vi "test_CalculateSpecificationBuildOrder.vi"() -> (3 "Pass?":bool)   [LabVIEW 2020, in "Tests.SolutionBuilder.lvlib"]
uses:
  Tests.SolutionBuilder.lvlib
  SolutionBuilder/SolutionBuilder.lvclass
  SolutionBuilder/ProjectItem/ProjectItem.lvclass
panel:
  out "test results":u32 format="%02b"
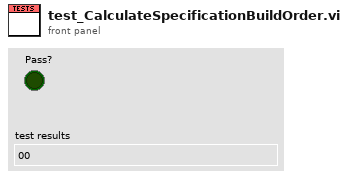
[diagram p1: front panel]
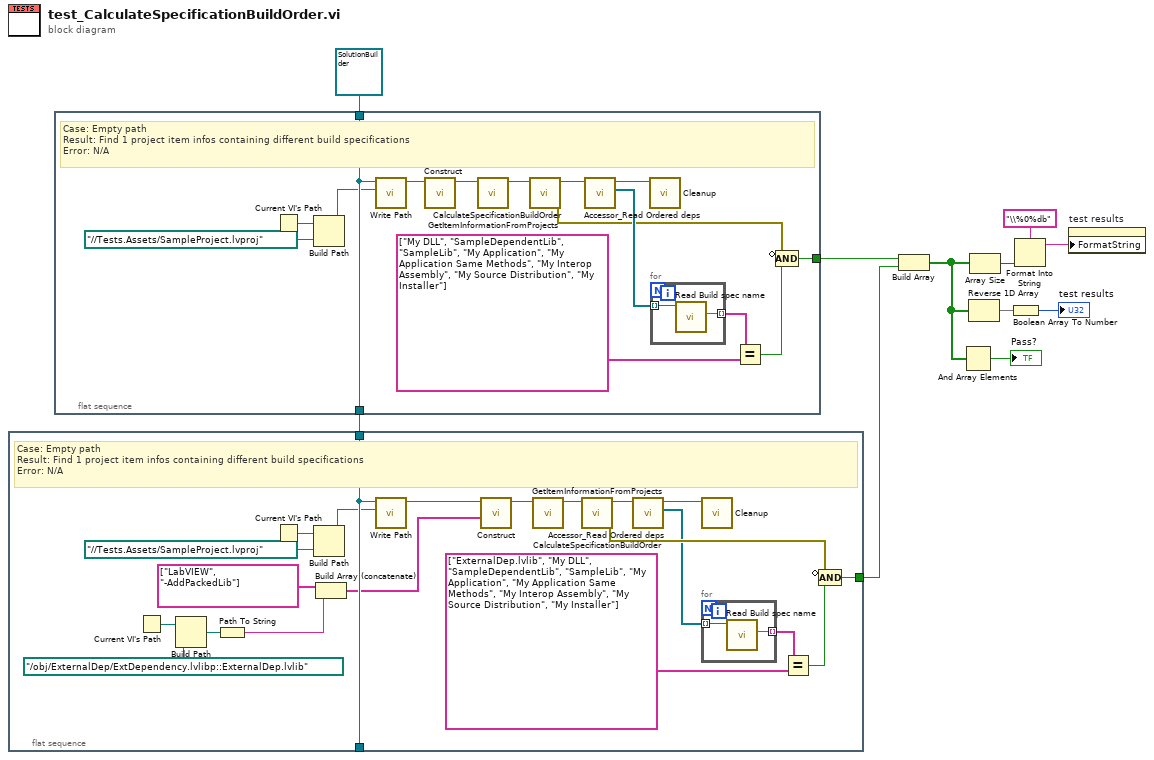
[diagram p0: block diagram]
diagram:
  n1 = flat-sequence {
    tunnel: [w28] -> w1
    tunnel: w2 -> [w32]
    tunnel: [w32] -> _
    frame #0 {
      # "Case: Empty path\nResult: Find 1 project item infos containing different build specifications\nError: N/A"
      n2 = Current VI's Path() -> (path=w21:path)
      n3 = Build Path(base path=w21, name or relative path=path "../obj/ExternalDep/ExtDependency.lvlibp::ExternalDep.lvlib" ("Path")) -> (appended path=w23:path)
      n4 = Path To String(path=w23) -> (string=w24:string)
      n5 = Current VI's Path() -> (path=w31:path)
      n6 = Build Path(base path=w31, name or relative path=path "../../Tests.Assets/SampleProject.lvproj" ("Path")) -> (appended path=w29:path)
      n7 = Build Array (concatenate)(string[] ["LabVIEW", "-AddPackedLib"] ("App.Args"), w24) -> (w22:string[])
      n8 = call-dynamic "Write Path.vi"("Path"=w29, "SolutionBuilder in"=w32) -> ("SolutionBuilder out"=w27:refnum<class "SolutionBuilder.lvclass">)  [unwired: 9 in]
      n9 = call-dynamic "Construct.vi"("App.Args"=w22, "SolutionBuilder in"=w27) -> ("SolutionBuilder out"=w19:refnum<class "SolutionBuilder.lvclass">)  [unwired: 8 in, 1 out]
      n10 = call-dynamic "GetItemInformationFromProjects.vi"("SolutionBuilder in"=w19) -> ("SolutionBuilder out"=w18:refnum<class "SolutionBuilder.lvclass">)  [unwired: 9 in, 1 out]
      n11 = call-dynamic "CalculateSpecificationBuildOrder.vi"("SolutionBuilder in"=w18) -> ("error out"=w15:errorcluster, "SolutionBuilder out"=w17:refnum<class "SolutionBuilder.lvclass">)  [unwired: 9 in]
      n12 = call "Accessor_Read Ordered deps.vi"("SolutionBuilder in"=w17) -> ("Ordered deps"=w14:refnum<class "ProjectItem.lvclass">[], "SolutionBuilder out"=w16:refnum<class "SolutionBuilder.lvclass">)  [unwired: 8 in, 1 out]
      n13 = call-dynamic "Cleanup.vi"("SolutionBuilder in"=w16) -> ()  [unwired: 9 in, 2 out]
      n14 = for {
        tunnel: w14 -> [w34] mode=indexing
        tunnel: [w33] -> w13 mode=indexing
        n15 = call-dynamic "Read Build spec name.vi"("ProjectItem in"=w34) -> ("Build spec name"=w33:string)  [unwired: 9 in, 1 out]
      }
      n16 = Equal?(x=w13, y=string[] ["ExternalDep.lvlib", "My DLL", "SampleDependentLib", "SampleLib", "My Application", "My Application Same Methods", "My Interop Assembly", "My Source Distribution", "My Installer"] ("Array")) -> (x = y?=w26:bool)
      n17 = Compound Arithmetic op=AND(invert w15, w26) -> (w28:bool)
    }
  }
  n18 = flat-sequence {
    tunnel: [w45] -> w5
    tunnel: refnum<class "SolutionBuilder.lvclass"> refnum ("SolutionBuilder in") -> [w49]
    tunnel: [w49] -> w2
    frame #0 {
      # "Case: Empty path\nResult: Find 1 project item infos containing different build specifications\nError: N/A"
      n19 = Current VI's Path() -> (path=w48:path)
      n20 = Build Path(base path=w48, name or relative path=path "../../Tests.Assets/SampleProject.lvproj" ("Path")) -> (appended path=w46:path)
      n21 = call-dynamic "Write Path.vi"("Path"=w46, "SolutionBuilder in"=w49) -> ("SolutionBuilder out"=w44:refnum<class "SolutionBuilder.lvclass">)  [unwired: 9 in]
      n22 = call-dynamic "Construct.vi"("SolutionBuilder in"=w44) -> ("SolutionBuilder out"=w42:refnum<class "SolutionBuilder.lvclass">)  [unwired: 9 in, 1 out]
      n23 = call-dynamic "GetItemInformationFromProjects.vi"("SolutionBuilder in"=w42) -> ("SolutionBuilder out"=w41:refnum<class "SolutionBuilder.lvclass">)  [unwired: 9 in, 1 out]
      n24 = call-dynamic "CalculateSpecificationBuildOrder.vi"("SolutionBuilder in"=w41) -> ("error out"=w37:errorcluster, "SolutionBuilder out"=w40:refnum<class "SolutionBuilder.lvclass">)  [unwired: 9 in]
      n25 = call "Accessor_Read Ordered deps.vi"("SolutionBuilder in"=w40) -> ("Ordered deps"=w38:refnum<class "ProjectItem.lvclass">[], "SolutionBuilder out"=w39:refnum<class "SolutionBuilder.lvclass">)  [unwired: 8 in, 1 out]
      n26 = call-dynamic "Cleanup.vi"("SolutionBuilder in"=w39) -> ()  [unwired: 9 in, 2 out]
      n27 = for {
        tunnel: w38 -> [w51] mode=indexing
        tunnel: [w50] -> w36 mode=indexing
        n28 = call-dynamic "Read Build spec name.vi"("ProjectItem in"=w51) -> ("Build spec name"=w50:string)  [unwired: 9 in, 1 out]
      }
      n29 = Equal?(x=w36, y=string[] ["My DLL", "SampleDependentLib", "SampleLib", "My Application", "My Application Same Methods", "My Interop Assembly", "My Source Distribution", "My Installer"] ("Array")) -> (x = y?=w43:bool)
      n30 = Compound Arithmetic op=AND(invert w37, w43) -> (w45:bool)
    }
  }
  n31 = Build Array(w5, w1) -> (w9:bool[])
  n32 = And Array Elements(Boolean array=w9) -> (logical AND=→"Pass?":bool)
  n33 = Reverse 1D Array(array=w9) -> (reversed array=w4:bool[])
  n34 = Array Size(array=w9) -> (size(s)=w7:i32)
  n35 = Boolean Array To Number(Boolean array=w4) -> (number=→"test results":u32)
  n36 = Format Into String(format string="\\%0%db", w7) -> (resulting string=w6:string)  [unwired: 2 in, 1 out]
  n37 = property on="test results" class="DigNum (strict)"("FormatString"=w6) -> ()  [unwired: 2 in, 2 out]
